vi "Parse Data.vi"(11 "read buffer":string) -> (3 "Numeric Control":dbl)   [LabVIEW 2015, in "HH802U.lvclass"]
uses:
  HH802U.lvclass
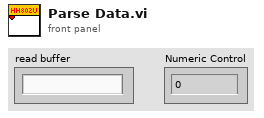
[diagram p1: front panel]
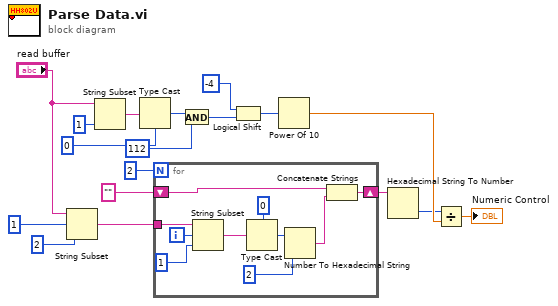
[diagram p0: block diagram]
diagram:
  n1 = String Subset(string="read buffer", offset (0)=1, length (rest)=2 ("length (rest)")) -> (substring=w4:string)
  n2 = String Subset(string="read buffer", length (rest)=1 ("length (rest)")) -> (substring=w8:string)  [unwired: 1 in]
  n3 = Type Cast(type=u8 0 ("byte count"), x=w8) -> (*(type *) &x=w11:u8)
  n4 = for {
    N: 2 -> [_]
    tunnel: w4 -> [w28]
    shift-right: [w21] -> w6
    shift-left: "" -> [w20]
    i -> [w27]
    n5 = String Subset(string=w28, offset (0)=w27, length (rest)=1 ("length (rest)")) -> (substring=w25:string)
    n6 = Type Cast(type=u8 0 ("byte count"), x=w25) -> (*(type *) &x=w22:u8)
    n7 = Number To Hexadecimal String(1:i16 2 ("width (-)"), 2:w22) -> (0:w19:string)
    n8 = Concatenate Strings(w20, w19) -> (w21:string)
  }
  n9 = And(x=w11, y=u8 112 ("*(type *) &x")) -> (x .and. y?=w14:u8)
  n10 = Logical Shift(y=i8 -4 ("x"), x=w14) -> (x << y=w16:u8)
  n11 = Power Of 10(x=w16) -> (10^x=w17:dbl)
  n12 = Hexadecimal String To Number(string=w6) -> (number=w15:u32)  [unwired: 2 in, 1 out]
  n13 = Divide(x=w15, y=w17) -> (x/y=→"Numeric Control":dbl)
